vi "SetLvClassPath.vi"(0 "ClassWriter":refnum<class "ClassWriter.lvclass">, 1 "ClassPath":path, 2 "ClassName":string, 5 "error in (no error)":errorcluster) -> (14 "ClassWriter":refnum<class "ClassWriter.lvclass">, 19 "error out":errorcluster)   [LabVIEW 2016, in "ClassWriter.lvclass"]
uses:
  <resource>/Framework/Providers/Open_GDS/ClassProviders/Provider_BaseClassInterface/ClassWriter_class/ClassWriter.lvclass
  <resource>/Framework/Providers/Open_GDS/ClassProviders/Provider_BaseClassInterface/ClassWriter_class/ClassWriter.lvclass/ClassWriter.ctl
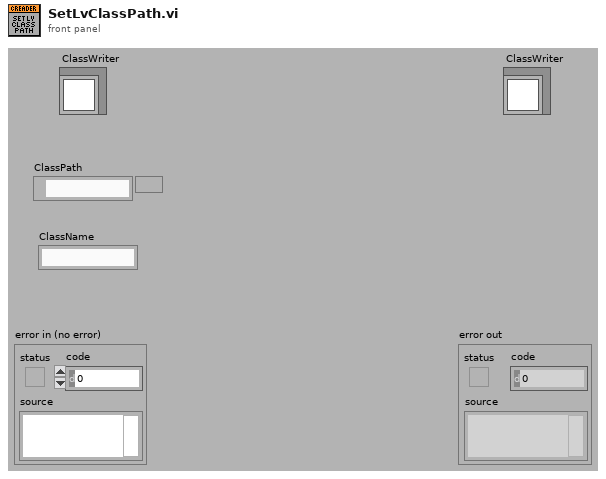
[diagram p1: front panel]
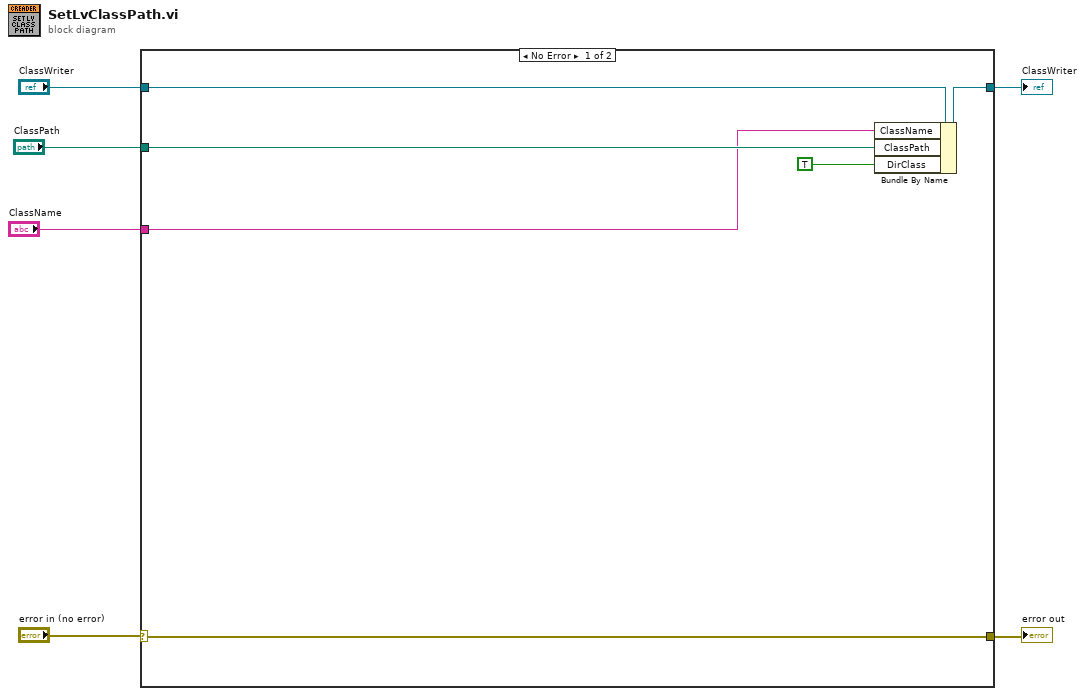
[diagram p0: block diagram]
diagram:
  n1 = case shown="No Error" "error in (no error)" {
    selector: "error in (no error)" -> [w10 w13]
    tunnel: "ClassWriter" -> [w12 w14]
    tunnel: [w11 w14] -> w5
    tunnel: [w10 w13] -> w3
    tunnel: "ClassPath" -> [w9 _]
    tunnel: "ClassName" -> [w7 _]
    frame No Error {
      n2 = Bundle By Name(cluster=w12, "ClassName"=w7, "ClassPath"=w9, "DirClass"=TRUE) -> (w11:refnum<class "ClassWriter.lvclass">)
    }
    frame Error {
    }
  }
  "ClassWriter" <- w5
  "error out" <- w3
